vi "Actor Core.vi"(8 "error in":errorcluster, 11 "RandomDataChart in":refnum<class "NumericCounter.lvclass">) -> (0 "error out":errorcluster, 3 "Actor out":refnum<class "Actor.lvclass">)   [LabVIEW 2015, in "TestActors.lvlib" / "NumericCounter.lvclass"]
doc: "(<B>Filename</B>: Actor Framework.lvlib:Actor.lvclass:Actor Core.vi)\n\nReceives messages to the actor, reacts to them, and initiates any error handling that may shut the actor down.\n\nDescendant classes may override this VI to append parallel tasks for the actor to complete while it handles messages. Overrides use the Call Parent Method node."
uses:
  NumericCounter.lvclass
  <vilib>/ActorFramework/Actor/Actor.lvclass
  IViewable/IViewable/IViewable.lvclass
panel:
  out "Count":i32 format="Count: %.0f"
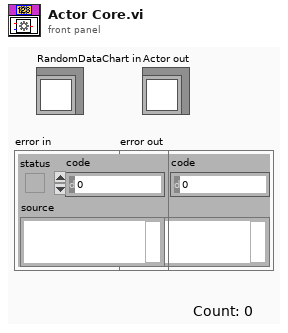
[diagram p1: front panel]
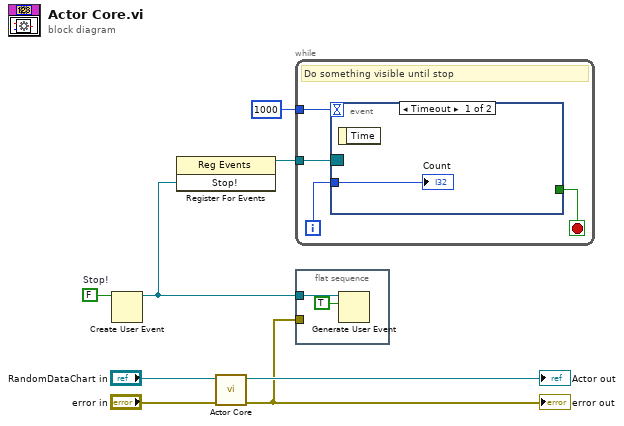
[diagram p0: block diagram]
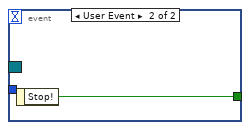
[diagram p2: hidden frame]
diagram:
  w5 = FALSE  # Stop!
  n1 = Create User Event(user event datatype=w5) -> (user event=w2:refnum<user-event>)  [unwired: 1 in, 1 out]
  n2 = register-events(w2) -> (reference out=w3:refnum<event-registration>)  [unwired: 2 in, 1 out]
  n3 = call-parent "Actor Core.vi"("error in"="error in", "IViewable In"="RandomDataChart in") -> ("error out"=w4:errorcluster, "Actor out"=→"Actor out":refnum<class "Actor.lvclass">)  [unwired: 8 in]
  "error out" <- w4
  n4 = while {
    tunnel: w3 -> [w12]
    tunnel: 1000 -> [w11]
    i -> [w9]
    stop <- w10 stop-if-true
    # "Do something visible until stop"
    n5 = event shown="[0] Timeout" {
      selector: w12 -> [_ _]
      dyn-events: _ -> [_ _]
      timeout: w11 -> [_ _]
      tunnel: [_ w14] -> w10
      tunnel: w9 -> [w13 _]
      event Timeout {
        n6 = event-data() -> ()  [unwired: 1 in, 1 out]
        "Count" <- w13
      }
      event User Event {
        n7 = event-data() -> ("Stop!"=w14:bool)  [unwired: 1 in]
      }
    }
  }
  n8 = flat-sequence {
    tunnel: w2 -> [w16]
    tunnel: w4 -> [_]
    frame #0 {
      n9 = Generate User Event(user event=w16, event data cluster=TRUE ("event data")) -> ()  [unwired: 2 in, 2 out]
    }
  }
